vi "콜라자판기(생산자소비자).vi"() -> ()   [LabVIEW 2014]
uses:
  Status.ctl
panel:
  out "Count Up":i32
  out "그림 링":u16(ring)
  in  "종료":bool
  in  "반환":bool
  in  "구매":bool
  out "투입금액":i32 format="%.0f원"
  in  "동전":T1
  # "콜라자판기"
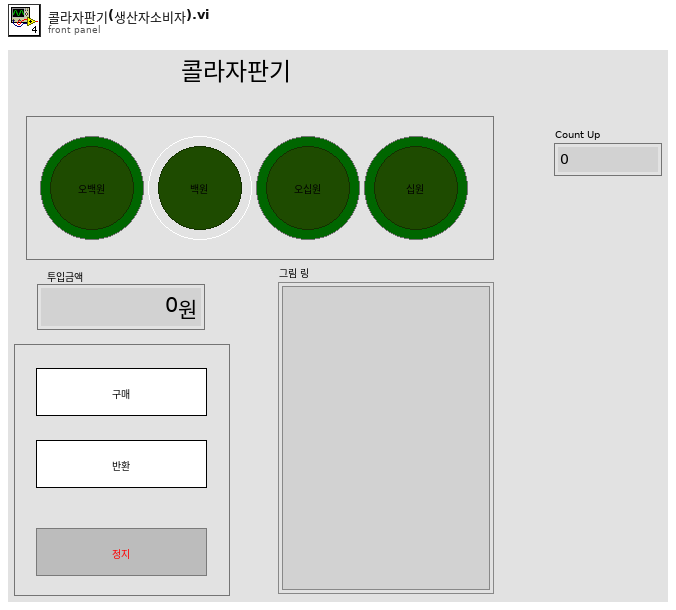
[diagram p1: front panel]
types:
  T1 = cluster{"불리언":bool, "불리언 2":bool, "불리언 3":bool, "불리언 4":bool}
  T2 = typedef "Status.ctl" = enum16{"Idle", "초기화", "종료", "구매", "반환", "기다림"}
  T3 = enum8{"Enabled", "Disabled", "Disabled and Grayed Out"}
  T4 = enum32{"invalid app kind", "Development System", "Run Time System", "Student Edition", "Embedded LabVIEW", "Evaluation", "Custom"}
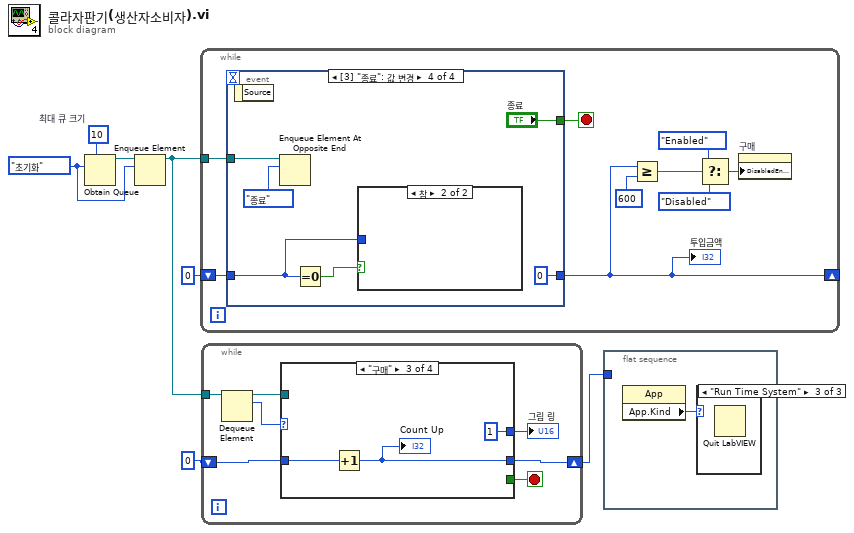
[diagram p0: block diagram]
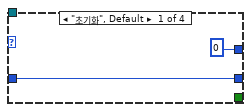
[diagram p4: hidden frame]
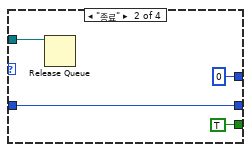
[diagram p5: hidden frame]
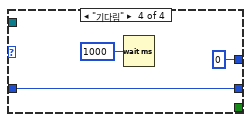
[diagram p6: hidden frame]
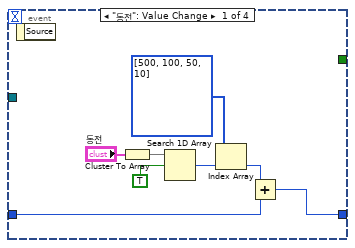
[diagram p7: hidden frame]
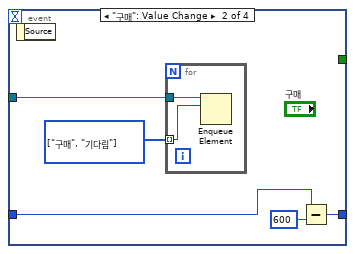
[diagram p8: hidden frame]
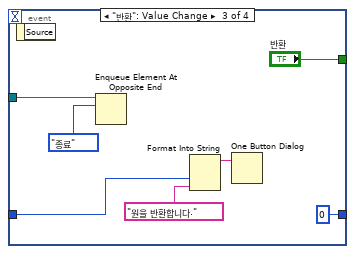
[diagram p9: hidden frame]
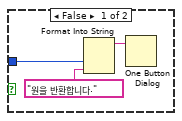
[diagram p10: hidden frame]
diagram:
  w4 = 10  # 최대 큐 크기
  w6 = Status."초기화" ("Status")
  n1 = Obtain Queue(max queue size (-1, unlimited)=w4, element data type=w6) -> (queue out=w7:refnum<queue>)  [unwired: 3 in, 2 out]
  n2 = Enqueue Element(queue=w7, element=w6) -> (queue out=w3:refnum<queue>)  [unwired: 2 in, 2 out]
  n3 = while {
    tunnel: w3 -> [w16]
    shift-right: [w9] -> _
    shift-left: 0 -> [w15]
    stop <- w8 stop-if-true
    n4 = event shown="[3] \"종료\": 값 변경" {
      selector: _ -> [_ _ _ _]
      dyn-events: _ -> [_ _ _ _]
      timeout: _ -> [_ _ _ _]
      tunnel: [w18 w29 0 0] -> w9
      tunnel: w16 -> [_ w27 w32 w43]
      tunnel: w15 -> [w17 w26 w35 w40]
      tunnel: [_ _ "반환" "종료"] -> w8
      event "동전": Value Change {
        n5 = event-data() -> ()  [unwired: 1 in, 1 out]
        n6 = Cluster To Array(cluster="동전") -> (array=w23:bool[])
        n7 = Search 1D Array(1D array=w23, element=TRUE) -> (index of element=w21:i32)  [unwired: 1 in]
        n8 = Index Array(array=i32[] [500, 100, 50, 10], index=w21) -> (element=w19:i32)
        n9 = Add(x=w19, y=w17) -> (x+y=w18:i32)
      }
      event "구매": Value Change {
        w25 = T2[] [enum."구매", enum."기다림"] items=["Idle", "초기화", "종료", "구매", "반환", "기다림"]
        n10 = event-data() -> ()  [unwired: 1 in, 1 out]
        n11 = for {
          tunnel: w27 -> [w31]
          tunnel: w25 -> [w30] mode=indexing
          n12 = Enqueue Element(queue=w31, element=w30) -> ()  [unwired: 2 in, 3 out]
        }
        n13 = Subtract(x=w26, y=600) -> (x-y=w29:i32)
      }
      event "반환": Value Change {
        n14 = event-data() -> ()  [unwired: 1 in, 1 out]
        n15 = Enqueue Element At Opposite End(queue=w32, element=Status."종료" ("Status")) -> ()  [unwired: 2 in, 3 out]
        n16 = Format Into String(w35, "원을 반환합니다.") -> (resulting string=w37:string)  [unwired: 3 in, 1 out]
        n17 = One Button Dialog(message=w37) -> ()  [unwired: 1 in, 1 out]
      }
      event "종료": Value Change {
        n18 = event-data() -> ()  [unwired: 1 in, 1 out]
        n19 = Enqueue Element At Opposite End(queue=w43, element=Status."종료" ("Status")) -> ()  [unwired: 2 in, 3 out]
        n20 = Equal To 0?(x=w40) -> (x = 0?=w41:bool)
        n21 = case shown="참" w41 {
          tunnel: w40 -> [w45 _]
          frame False {
            n22 = Format Into String(w45, "원을 반환합니다.") -> (resulting string=w47:string)  [unwired: 3 in, 1 out]
            n23 = One Button Dialog(message=w47) -> ()  [unwired: 1 in, 1 out]
          }
          frame True {
          }
        }
      }
    }
    "투입금액" <- w9
    n24 = Greater Or Equal?(x=w9, y=600) -> (x >= y?=w13:bool)
    n25 = Select(t=T3."Enabled" ("비활성화"), s=w13, f=T3."Disabled" ("비활성화")) -> (s? t:f=w10:T3)
    n26 = property on="구매" class="Bool"("DisabledEnum"=w10) -> ()  [unwired: 2 in, 2 out]
  }
  n27 = while {
    tunnel: w3 -> [w54]
    shift-right: [w48] -> w1
    shift-left: 0 -> [w49]
    stop <- w51 stop-if-true
    n28 = Dequeue Element(queue=w54) -> (queue out=w50:refnum<queue>, element=w53:T2)  [unwired: 2 in, 2 out]
    n29 = case shown="\"구매\"" w53 {
      tunnel: [u16 0 u16 0 u16 1 u16 0] -> w52
      tunnel: [_ TRUE _ _] -> w51
      tunnel: w50 -> [_ w59 _ _]
      tunnel: w49 -> [w55 w57 w62 w64]
      tunnel: [w55 w57 w61 w64] -> w48
      frame "초기화", Default {
      }
      frame "종료" {
        n30 = Release Queue(queue=w59) -> ()  [unwired: 2 in, 3 out]
      }
      frame "구매" {
        n31 = Increment(x=w62) -> (x+1=w61:i32)
        "Count Up" <- w61
      }
      frame "기다림" {
        n32 = Wait (ms)(milliseconds to wait=u32 1000 ("대기 시간(ms)")) -> ()  [unwired: 1 out]
      }
    }
    "그림 링" <- w52
  }
  n33 = flat-sequence {
    tunnel: w1 -> [_]
    frame #0 {
      n34 = property class="App"() -> ("App.Kind"=w67:T4)  [unwired: 2 in, 2 out]
      n35 = case shown="\"Run Time System\"" w67 {
        frame "invalid app kind", Default {
        }
        frame "Development System" {
        }
        frame "Run Time System" {
          n36 = Quit LabVIEW() -> ()  [unwired: 1 in]
        }
      }
    }
  }
